vi "Measure Resistance Only_ERMod.vi"(6 "Published_ID":string="_Free", 7 "Settings":T2 {"Sense" items=["Local"=1008, "Remote"=1009]}, 8 "error in (no error)":errorcluster, 9 "current level":dbl format="%_6p", 10 "Pins":string[](array[string]), 11 "Semiconductor Module Context":T3) -> (0 "error out":errorcluster, 3 "Semiconductor Module Context Out":T3)   [LabVIEW 2013]
uses:
  <vilib>/NI_TestStand_SemiconductorModule/NI_TestStand_Semiconductor_Module.lvlibp/PinMap/General/SemiconductorModuleContext.ctl
  <instrlib>/niDCPower/nidcpower.llb/niDCPower Sense.ctl
  <instrlib>/niDCPower/nidcpower.llb/niDCPower Wait For Event - Event.ctl
  <vilib>/NI_TestStand_SemiconductorModule/NI_TestStand_Semiconductor_Module.lvlibp/PinMap/DC Power/PinsToNIDCPowerSessions.vi
  <vilib>/NI_TestStand_SemiconductorModule/NI_TestStand_Semiconductor_Module.lvlibp/PinMap/General/Publish/PublishDataDoubleFunctionalTest.vi
  <vilib>/NI_TestStand_SemiconductorModule/NI_TestStand_Semiconductor_Module.lvlibp
panel:
  out "R Array":dbl[](array[numeric])
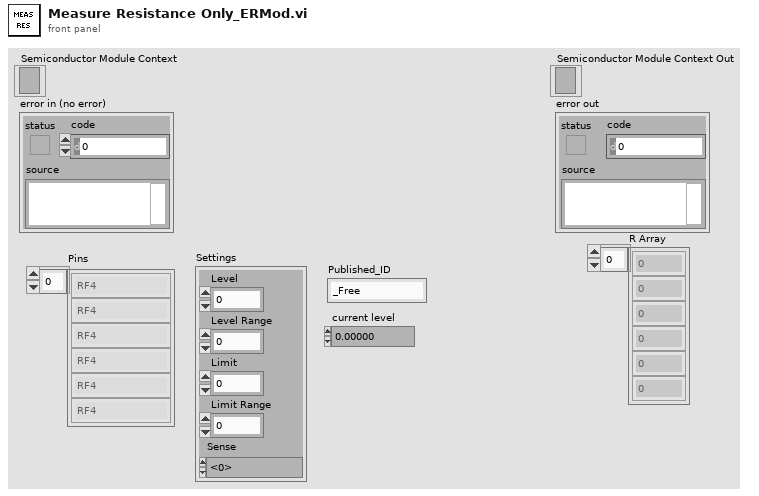
[diagram p1: front panel]
types:
  T1 = typedef "niDCPower Sense.ctl" = i32
  T2 = cluster{"Level":dbl, "Level Range":dbl, "Limit":dbl, "Limit Range":dbl, "Sense":T1}
  T3 = typedef "NI_TestStand_Semiconductor_Module.lvlibp/SemiconductorModuleContext.ctl" = refnum<k7>
  T4 = typedef "niDCPower Wait For Event - Event.ctl" = i32
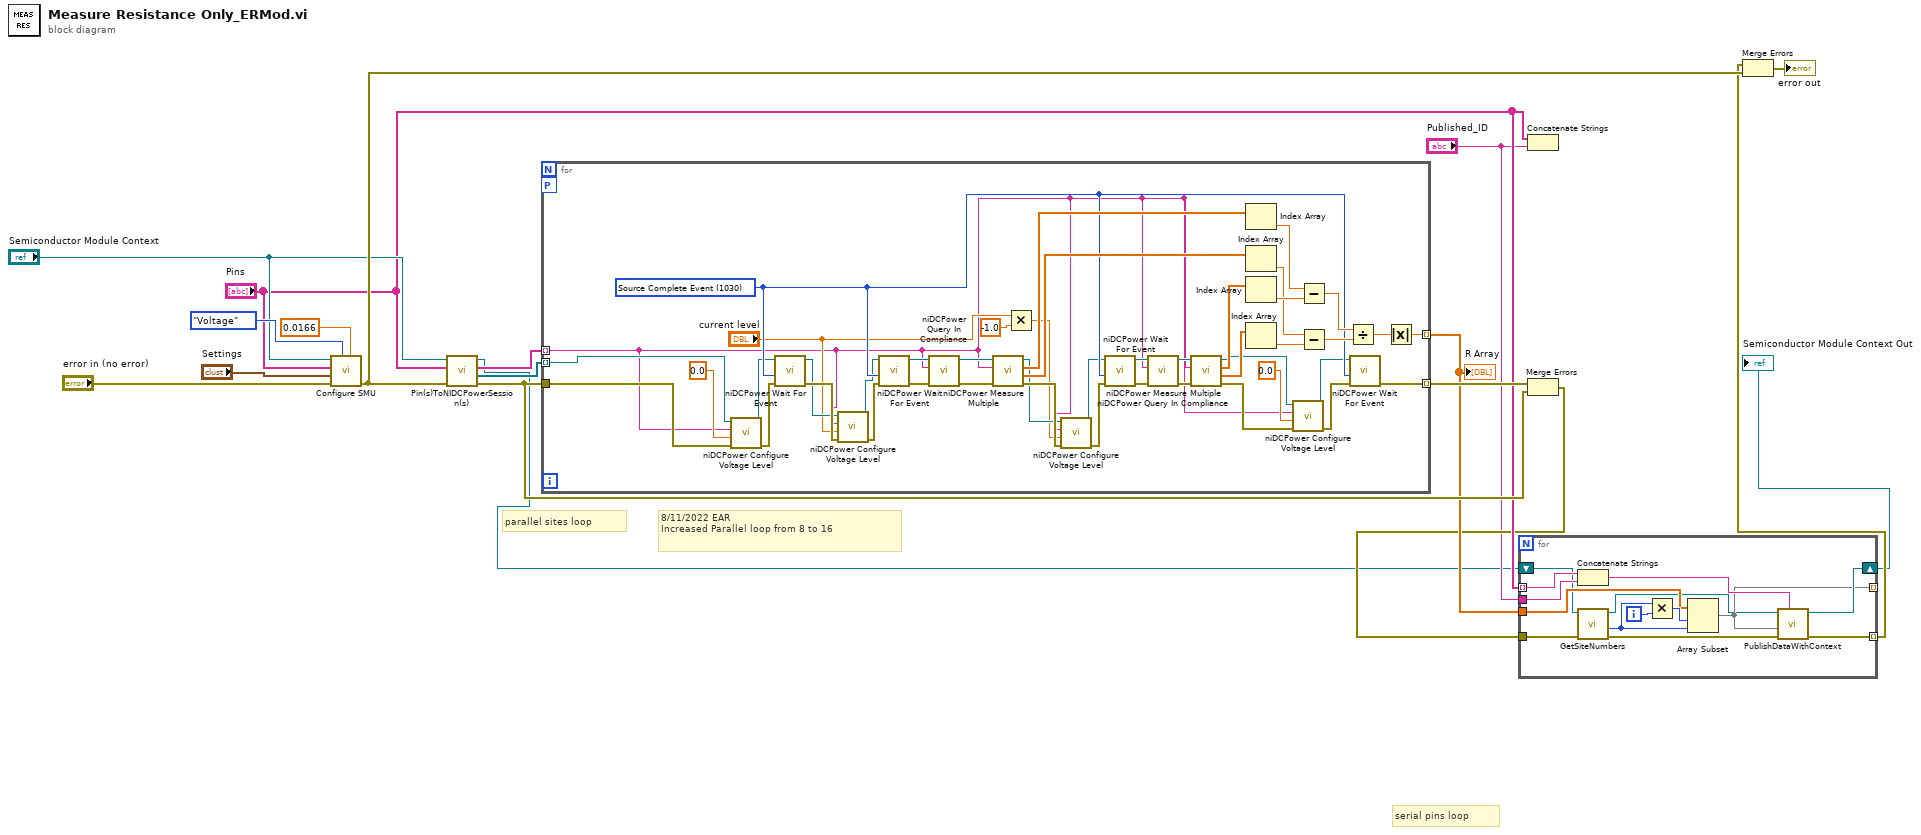
[diagram p0: block diagram]
diagram:
  # "8/11/2022 EAR\nIncreased Parallel loop from 8 to 16"
  # "parallel sites loop"
  # "serial pins loop"
  n1 = call "Configure SMU.vi"("aperture time"=0.0166, "Source Mode"=enum16{"Voltage", "Current"}."Voltage", "error in (no error)"="error in (no error)", "Settings"="Settings", "Pins"="Pins", "Semiconductor Module Context"="Semiconductor Module Context") -> ("error out"=w16:errorcluster)  [unwired: 5 in]
  n2 = call-poly <vilib>:"Pin(s)ToNIDCPowerSession(s).vi"("error in (no error)"=w16, "Pins"="Pins", "Semiconductor Module Context"="Semiconductor Module Context") -> ("error out"=w8:errorcluster, "Instrument Sessions"=w10:refnum<k15>[], "Channel Lists"=w11:string[], "Semiconductor Module Context Out"=w2:T3)  [unwired: 4 in, 1 out]
  n3 = for {
    tunnel: w11 -> [w19] mode=indexing
    tunnel: w10 -> [w36] mode=indexing
    workers-P: _ -> [_]
    tunnel: w8 -> [w39]
    tunnel: [w61] -> w9 mode=indexing
    tunnel: [w54] -> w7 mode=indexing
    w40 = T4 1030 items=["Source Complete Event"=1030, "Measure Complete Event"=1031, "Sequence Iteration Complete Event"=1032, "Sequence Engine Done Event"=1033, "Pulse Complete Event"=1051, "Ready For Pulse Trigger Event"=1052] ("event")
    n4 = call <instrlib>:"niDCPower Configure Voltage Level.vi"("error in (no error)"=w39, "voltage level"=0.0 ("current level"), "channel name"=w19, "instrument handle"=w36) -> ("error out"=w38:errorcluster, "instrument handle out"=w37:refnum<k15>)  [unwired: 6 in]
    n5 = call <instrlib>:"niDCPower Wait For Event.vi"("error in (no error)"=w38, "event"=w40, "instrument handle"=w37) -> ("error out"=w34:errorcluster, "instrument handle out"=w31:refnum<k15>)  [unwired: 7 in]
    n6 = call <instrlib>:"niDCPower Configure Voltage Level.vi"("error in (no error)"=w34, "voltage level"="current level", "channel name"=w19, "instrument handle"=w31) -> ("error out"=w33:errorcluster, "instrument handle out"=w32:refnum<k15>)  [unwired: 6 in]
    n7 = call <instrlib>:"niDCPower Wait For Event.vi"("error in (no error)"=w33, "event"=w40, "instrument handle"=w32) -> ("error out"=w62:errorcluster, "instrument handle out"=w60:refnum<k15>)  [unwired: 7 in]
    n8 = call <instrlib>:"niDCPower Query In Compliance.vi"("error in (no error)"=w62, "channel name"=w19, "instrument handle"=w60) -> ("error out"=w58:errorcluster, "instrument handle out"=w59:refnum<k15>)  [unwired: 6 in, 1 out]
    n9 = call <instrlib>:"niDCPower Measure Multiple.vi"("error in (no error)"=w58, "channel name"=w19, "instrument handle"=w59) -> ("error out"=w29:errorcluster, "current measurements"=w55:dbl[], "voltage measurements"=w56:dbl[], "instrument handle out"=w26:refnum<k15>)  [unwired: 5 in]
    n10 = Multiply(x="current level", y=-1.0) -> (x*y=w25:dbl)
    n11 = call <instrlib>:"niDCPower Configure Voltage Level.vi"("error in (no error)"=w29, "voltage level"=w25, "channel name"=w19, "instrument handle"=w26) -> ("error out"=w28:errorcluster, "instrument handle out"=w27:refnum<k15>)  [unwired: 6 in]
    n12 = call <instrlib>:"niDCPower Wait For Event.vi"("error in (no error)"=w28, "event"=w40, "instrument handle"=w27) -> ("error out"=w49:errorcluster, "instrument handle out"=w52:refnum<k15>)  [unwired: 7 in]
    n13 = call <instrlib>:"niDCPower Query In Compliance.vi"("error in (no error)"=w49, "channel name"=w19, "instrument handle"=w52) -> ("error out"=w50:errorcluster, "instrument handle out"=w51:refnum<k15>)  [unwired: 6 in, 1 out]
    n14 = call <instrlib>:"niDCPower Measure Multiple.vi"("error in (no error)"=w50, "channel name"=w19, "instrument handle"=w51) -> ("error out"=w22:errorcluster, "current measurements"=w47:dbl[], "voltage measurements"=w48:dbl[], "instrument handle out"=w21:refnum<k15>)  [unwired: 5 in]
    n15 = Index Array(array=w56) -> (element=w46:dbl)  [unwired: 1 in]
    n16 = Index Array(array=w55) -> (element=w44:dbl)  [unwired: 1 in]
    n17 = Index Array(array=w48) -> (element=w45:dbl)  [unwired: 1 in]
    n18 = Index Array(array=w47) -> (element=w43:dbl)  [unwired: 1 in]
    n19 = call <instrlib>:"niDCPower Configure Voltage Level.vi"("error in (no error)"=w22, "voltage level"=0.0 ("current level"), "channel name"=w19, "instrument handle"=w21) -> ("error out"=w24:errorcluster, "instrument handle out"=w23:refnum<k15>)  [unwired: 6 in]
    n20 = Subtract(x=w46, y=w45) -> (x-y=w42:dbl)
    n21 = Subtract(x=w44, y=w43) -> (x-y=w41:dbl)
    n22 = Divide(x=w42, y=w41) -> (x/y=w57:dbl)
    n23 = call <instrlib>:"niDCPower Wait For Event.vi"("error in (no error)"=w24, "event"=w40, "instrument handle"=w23) -> ("error out"=w61:errorcluster)  [unwired: 7 in, 1 out]
    n24 = Absolute Value(x=w57) -> (abs(x)=w54:dbl)
  }
  "R Array" <- w7
  n25 = Concatenate Strings("Pins", "Published_ID") -> ()  [unwired: 1 out]
  n26 = Merge Errors(w9, w8) -> (w5:errorcluster)
  n27 = for {
    tunnel: [w71] -> w4 mode=indexing
    tunnel: "Pins" -> [w75] mode=indexing
    tunnel: w7 -> [w72]
    tunnel: "Published_ID" -> [w74]
    shift-right: [w69] -> w1
    shift-left: w2 -> [w66]
    tunnel: [w68] -> _ mode=indexing
    tunnel: w5 -> [w63]
    i -> [w76]
    n28 = Concatenate Strings(w75, w74) -> (w70:string)
    n29 = call <vilib>:"GetSiteNumbers.vi"("error in (no error)"=w63, "Semiconductor Module Context"=w66) -> ("error out"=w67:errorcluster, "Number Of Sites"=w64:i32, "Semiconductor Module Context Out"=w65:T3)  [unwired: 6 in, 1 out]
    n30 = Multiply(x=w64, y=w76) -> (x*y=w73:i32)
    n31 = Array Subset(array=w72, index=w73, length=w64) -> (w68:dbl[])
    n32 = call-poly <vilib>:"PublishDataWithContext.vi"("Published Data Id"=w70, "error in (no error)"=w67, "Data In"=w68, "Semiconductor Module Context"=w65) -> ("error out"=w71:errorcluster, "Semiconductor Module Context Out"=w69:T3)  [unwired: 6 in]
  }
  "Semiconductor Module Context Out" <- w1
  n33 = Merge Errors(w4, w16) -> (→"error out":errorcluster)
